vi "ArmSetTargetText.vi"(9 "TargetGamePiece":string, 11 "TargetArmPosition":string) -> ()   [LabVIEW 2023]
uses:
  ArmGlobal.vi
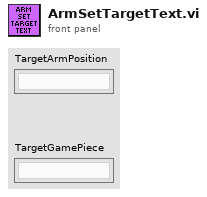
[diagram p1: front panel]
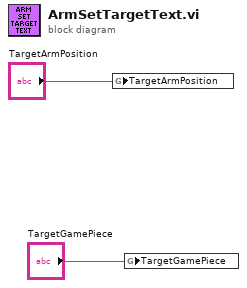
[diagram p0: block diagram]
diagram:
  n1 = global write "ArmGlobal.vi" "TargetArmPosition"("TargetArmPosition") -> ()
  n2 = global write "ArmGlobal.vi" "TargetGamePiece"("TargetGamePiece") -> ()
